vi "sub_hasWinningMove.vi"(9 "player":string, 11 "array":string[](array[string])) -> (1 "winning move":i32, 3 "has winning move":bool)   [LabVIEW 2018]
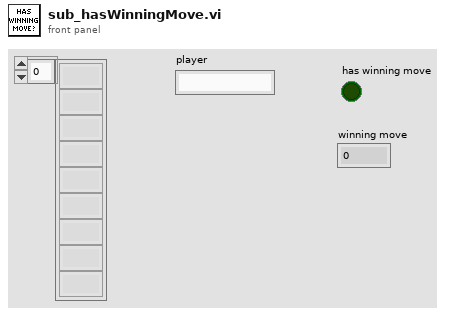
[diagram p1: front panel]
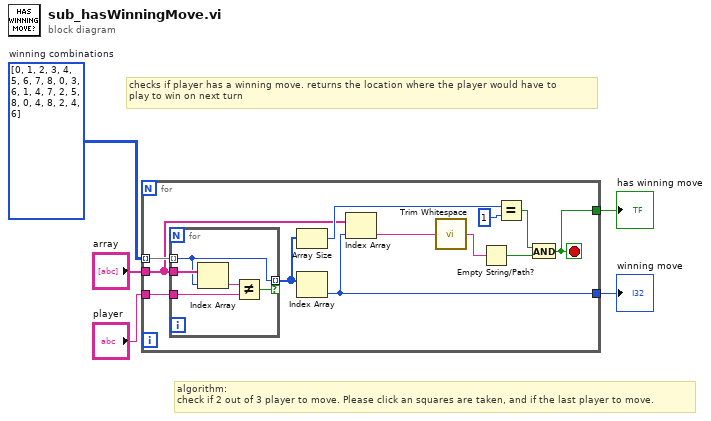
[diagram p0: block diagram]
diagram:
  w4 = i32[][] [[0, 1, 2], [3, 4, 5], [6, 7, 8], [0, 3, 6], [1, 4, 7], [2, 5, 8], [0, 4, 8], [2, 4, 6]]  # winning combinations
  # "algorithm:\ncheck if 2 out of 3 player to move. Please click an squares are taken, and if the last player to move."
  # "checks if player has a winning move. returns the location where the player would have to\nplay to win on next turn"
  n1 = for {
    tunnel: "array" -> [w12]
    tunnel: w4 -> [w17] mode=indexing
    tunnel: "player" -> [w16]
    tunnel: [w7] -> w2
    tunnel: [w6] -> w1
    stop <- w6 stop-if-true
    n2 = for {
      tunnel: w12 -> [w22]
      tunnel: w17 -> [w20] mode=indexing
      tunnel: w16 -> [w21]
      tunnel: [w20] -> w13 mode=indexing if=w18
      n3 = Index Array(array=w22, index=w20) -> (element=w19:string)
      n4 = Not Equal?(x=w19, y=w21) -> (x != y?=w18:bool)
    }
    n5 = Array Size(array=w13) -> (size(s)=w15:i32)
    n6 = Index Array(array=w13) -> (element=w7:i32)  [unwired: 1 in]
    n7 = Index Array(array=w12, index=w7) -> (element=w11:string)
    n8 = call <vilib>:"Trim Whitespace.vi"("string"=w11) -> ("trimmed string"=w10:string)  [unwired: 1 in]
    n9 = Empty String/Path?(string/path=w10) -> (empty?=w9:bool)
    n10 = Equal?(x=w15, y=1) -> (x = y?=w8:bool)
    n11 = And(x=w8, y=w9) -> (x .and. y?=w6:bool)
  }
  "has winning move" <- w1
  "winning move" <- w2
